vi "GetAllStationList.vi"(8 "Error In":errorcluster) -> (0 "Error Out":errorcluster, 2 "Station":string[](array[string]))   [LabVIEW 2020]
uses:
  <vilib>/Utility/miscctls.llb/LVRowAndColumnUnsignedTypeDef.ctl
  <vilib>/httpClient/LabVIEWHTTPClient.lvlib
  user32.dll
panel:
  in  "Close":bool
  out "TitleBar":bool
  in  "Select":bool
  in  "Stations":i32(listbox)
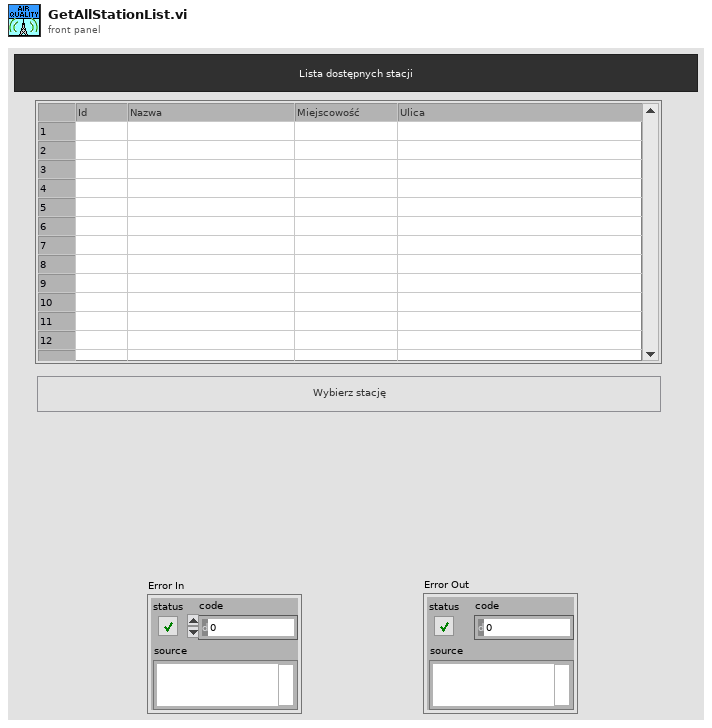
[diagram p1: front panel]
types:
  T1 = enum32{"Invalid", "Standard", "Closed", "Hidden", "Minimized", "Maximized"}
  T2 = cluster{"id":dbl, "stationName":string, "gegrLat":string, "gegrLon":string, "city":cluster{"id":dbl, "name":string, "commune":cluster{"communeName":string, "districtName":string, "provinceName":string}}, "addressStreet":string}[]
  T3 = typedef "LVRowAndColumnUnsignedTypeDef.ctl" = cluster{"Row":u32, "Column":u32}
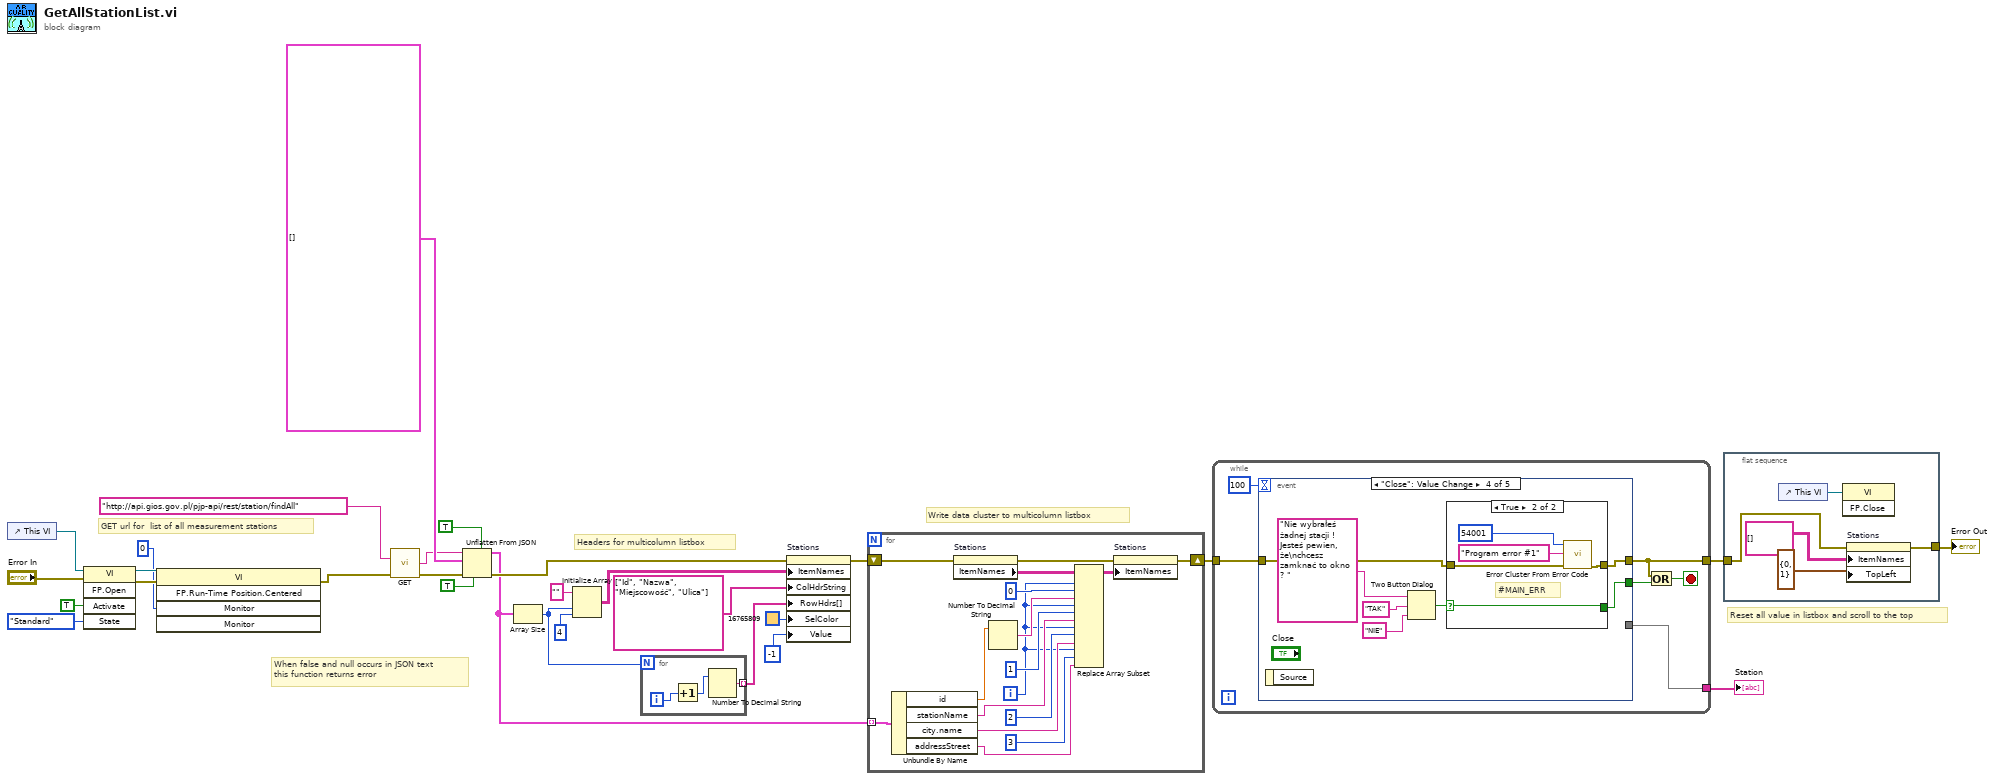
[diagram p0: block diagram]
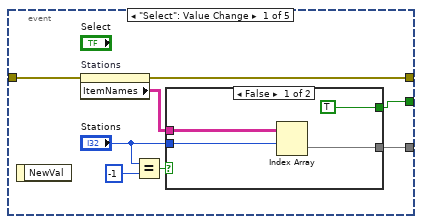
[diagram p2: hidden frame]
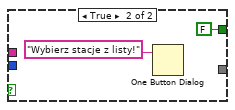
[diagram p3: hidden frame]
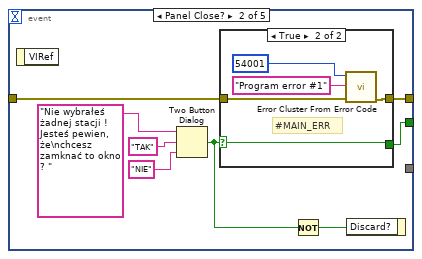
[diagram p4: hidden frame]
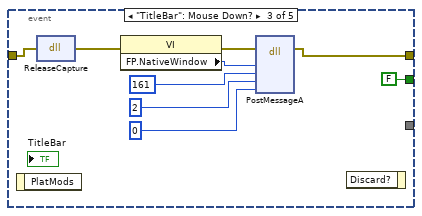
[diagram p6: hidden frame]
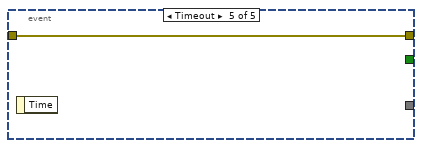
[diagram p8: hidden frame]
diagram:
  # "Reset all value in listbox and scroll to the top"
  # "When false and null occurs in JSON text\nthis function returns error"
  # "Write data cluster to multicolumn listbox"
  # "Headers for multicolumn listbox"
  # "GET url for  list of all measurement stations"
  n1 = control-ref of="This VI"() -> (w11:refnum<vi>)
  n2 = invoke class="VI" method="FP.Open"(reference=w11, error in="Error In", "Activate"=TRUE ("Activate?"), "State"=T1."Standard") -> (reference out=w3:refnum<vi>, error out=w4:errorcluster)  [unwired: 1 in, 3 out]
  n3 = invoke class="VI" method="FP.Run-Time Position.Centered"(reference=w3, error in=w4, "Monitor"=i16 0) -> (error out=w2:errorcluster)  [unwired: 2 in, 4 out]
  n4 = call <vilib>:"GET.vi"("url"="http://api.gios.gov.pl/pjp-api/rest/station/findAll", "error in (no error)"=w2) -> ("body"=w27:string, "error out"=w25:errorcluster)  [unwired: 10 in, 2 out]
  n5 = Unflatten From JSON(enable LabVIEW extensions? (T)=TRUE, JSON string=w27, type and defaults=T2 [], default null elements? (F)=TRUE, error in (no error)=w25) -> (value=w22:T2, error out=w24:errorcluster)  [unwired: 2 in]
  n6 = Array Size(array=w22) -> (size(s)=w16:i32)
  n7 = Initialize Array("", w16, 4 ("dimension size")) -> (w20:string[][])
  n8 = for {
    N: w16 -> [_]
    tunnel: [w30] -> w17 mode=indexing
    i -> [w32]
    n9 = Increment(x=w32) -> (x+1=w31:i32)
    n10 = Number To Decimal String(number=w31) -> (decimal integer string=w30:string)  [unwired: 1 in]
  }
  n11 = property on="Stations" class="MCListbox (strict)"(error in=w24, "ItemNames"=w20, "ColHdrString"=string[] ["Id", "Nazwa", "Miejscowość", "Ulica"] ("Column Header Strings[]"), "RowHdrs[]"=w17, "SelColor"=u32 16765809 ("Selection Color"), "Value"=-1 ("Stations")) -> (error out=w23:errorcluster)  [unwired: 1 in, 1 out]
  n12 = for {
    tunnel: w22 -> [w43] mode=indexing
    shift-right: [w45] -> w15
    shift-left: w23 -> [w48]
    i -> [w34]
    n13 = Unbundle By Name(w43) -> ("id"=w42:dbl, "stationName"=w37:string, "city.name"=w36:string, "addressStreet"=w33:string)
    n14 = property on="Stations" class="MCListbox (strict)"(error in=w48) -> (error out=w44:errorcluster, "ItemNames"=w47:string[][])  [unwired: 1 in, 1 out]
    n15 = Number To Decimal String(number=w42) -> (decimal integer string=w38:string)  [unwired: 1 in]
    n16 = Replace Array Subset(array=w47, new element #1=w38, index (row) #1=w34, index (col) #1=0 ("disabled index (col)"), new element #2=w37, index (row) #2=w34, index (col) #2=1 ("disabled index (col)"), new element #3=w36, index (row) #3=w34, index (col) #3=2 ("disabled index (col)"), new element #4=w33, index (row) #4=w34, index (col) #4=3 ("disabled index (row)")) -> (w46:string[][])
    n17 = property on="Stations" class="MCListbox (strict)"(error in=w44, "ItemNames"=w46) -> (error out=w45:errorcluster)  [unwired: 1 in, 1 out]
  }
  n18 = while {
    tunnel: w15 -> [w54]
    tunnel: [w50] -> w6
    tunnel: [w49] -> w12
    stop <- w51 stop-if-true
    n19 = event shown="[3] \"Close\": Value Change" {
      selector: _ -> [_ _ _ _ _]
      dyn-events: _ -> [_ _ _ _ _]
      timeout: 100 -> [_ _ _ _ _]
      tunnel: w54 -> [w62 w70 w85 w96 w107]
      tunnel: [w55 w71 FALSE w94 _] -> w53
      tunnel: [w61 w69 w84 w93 w107] -> w50
      tunnel: [w59 _ _ _ _] -> w49
      event "Select": Value Change {
        n20 = event-data() -> ()  [unwired: 1 in, 1 out]
        n21 = property on="Stations" class="MCListbox (strict)"(error in=w62) -> (error out=w61:errorcluster, "ItemNames"=w60:string[][])  [unwired: 1 in, 1 out]
        n22 = Equal?(x="Stations", y=-1) -> (x = y?=w58:bool)
        n23 = case shown="False" w58 {
          tunnel: w60 -> [w66 _]
          tunnel: [w65 _] -> w59
          tunnel: "Stations" -> [w64 _]
          tunnel: [TRUE FALSE] -> w55
          frame False {
            n24 = Index Array(array=w66, index (row)=w64) -> (element=w65:string[])  [unwired: 1 in]
          }
          frame True {
            n25 = One Button Dialog(message="Wybierz stacje z listy!") -> ()  [unwired: 1 in, 1 out]
          }
        }
      }
      event Panel Close? {
        n26 = event-data() -> ()  [unwired: 1 in, 1 out]
        n27 = Two Button Dialog(message="Nie wybrałeś żadnej stacji ! Jesteś pewien, że\nchcesz zamknać to okno ? ", 1:"NIE" ("F button name (\"Cancel\")"), 2:"TAK" ("message")) -> (T button?=w72:bool)
        n28 = case shown="True" w72 {
          selector: w72 -> [w78 w83]
          tunnel: [w78 w83] -> w71
          tunnel: w70 -> [w77 w82]
          tunnel: [w77 w81] -> w69
          frame False {
          }
          frame True {
            # "#MAIN_ERR"
            n29 = call <vilib>:"Error Cluster From Error Code.vi"("error in (no error)"=w82, "error message (\"\")"="Program error #1" ("error message (\"\")"), "error code (0)"=54001) -> ("error out"=w81:errorcluster)  [unwired: 6 in]
          }
        }
        n30 = Not(x=w72) -> (.not. x?=w73:bool)
        n31 = event-data("Discard?"=w73) -> ()  [unwired: 1 in, 1 out]
      }
      event "TitleBar": Mouse Down? {
        n32 = event-data() -> ()  [unwired: 1 in, 1 out]
        n33 = dll-call lib="user32.dll" fn="ReleaseCapture"(error in=w85) -> (error out=w89:errorcluster)  [unwired: 3 in, 1 out]
        n34 = property class="VI"(error in=w89) -> (error out=w90:errorcluster, "FP.NativeWindow"=w91:u64)  [unwired: 1 in, 1 out]
        n35 = dll-call lib="user32.dll" fn="PostMessageA"(error in=w90, "hWnd"=w91, "Msg"=161, "wParam"=2, "lParam"=0) -> (error out=w84:errorcluster)  [unwired: 7 in, 1 out]
        n36 = event-data() -> ()  [unwired: 2 in, 1 out]
      }
      event "Close": Value Change {
        n37 = event-data() -> ()  [unwired: 1 in, 1 out]
        n38 = Two Button Dialog(message="Nie wybrałeś żadnej stacji ! Jesteś pewien, że\nchcesz zamknać to okno ? ", 1:"NIE" ("F button name (\"Cancel\")"), 2:"TAK" ("message")) -> (T button?=w97:bool)
        n39 = case shown="True" w97 {
          selector: w97 -> [w101 w106]
          tunnel: [w101 w106] -> w94
          tunnel: w96 -> [w100 w105]
          tunnel: [w100 w104] -> w93
          frame False {
          }
          frame True {
            # "#MAIN_ERR"
            n40 = call <vilib>:"Error Cluster From Error Code.vi"("error in (no error)"=w105, "error message (\"\")"="Program error #1" ("error message (\"\")"), "error code (0)"=54001) -> ("error out"=w104:errorcluster)  [unwired: 6 in]
          }
        }
      }
      event Timeout {
        n41 = event-data() -> ()  [unwired: 1 in, 1 out]
      }
    }
    n42 = Or(x=w50, y=w53) -> (x .or. y?=w51:bool)
  }
  "Station" <- w12
  n43 = flat-sequence {
    tunnel: w6 -> [w111]
    tunnel: [w110] -> w5
    frame #0 {
      n44 = control-ref of="This VI"() -> (w112:refnum<vi>)
      n45 = invoke class="VI" method="FP.Close"(reference=w112) -> ()  [unwired: 2 in, 3 out]
      n46 = property on="Stations" class="MCListbox (strict)"(error in=w111, "ItemNames"=string[][] [] ("Item Names"), "TopLeft"=T3 {"Row"=0, "Column"=1} ("Top Left Visible Cell")) -> (error out=w110:errorcluster)  [unwired: 1 in, 1 out]
    }
  }
  "Error Out" <- w5
